vi "create buffer exchange.vi"(6 "FIFO modes (polling)":T2, 8 "error in":errorcluster, 10 "buffer count":u16, 11 "initial data table":T3) -> (0 "error out":errorcluster, 2 "consumer":T1, 3 "producer":T1)   [LabVIEW 2013, in "tag bus buffer exchange.lvlib"]
uses:
  tag bus buffer exchange.lvlib
  table/data table.ctl
  buffer exchange.ctl
  buffer reference.ctl
  table/data table.lvlib
  tag bus.lvlib
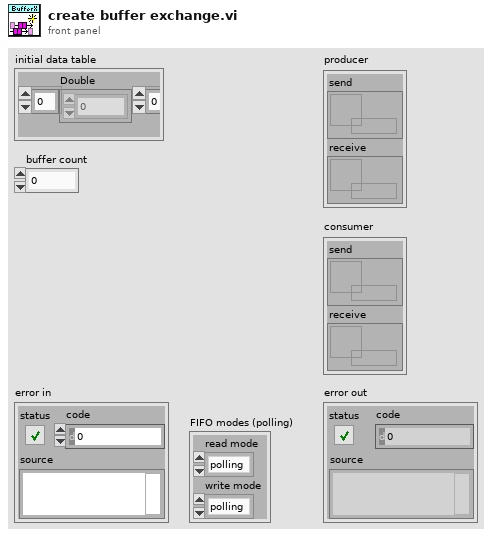
[diagram p1: front panel]
types:
  T1 = typedef "tag bus buffer exchange.lvlib/buffer exchange.ctl" = cluster{"send":refnum<k33>, "receive":refnum<k33>}
  T2 = cluster{"read mode":enum16{"polling", "blocking"}, "write mode":enum16{"polling", "blocking"}}
  T3 = typedef "tag bus.lvlib/data table.lvlib/data table.ctl" = cluster{"Double":dbl[], "Single":sgl[], "I64":i64[], "I32":i32[], "I16":i16[], "I8":i8[], "U64":u64[], "U32":u32[], "U16":u16[], "U8":u8[], "Boolean":bool[], "String":string[], "Array of Double":cluster{"DBL Array":dbl[]}[], "Array of Single":cluster{"SGL Array":sgl[]}[], "Array of I64":cluster{"I64 Array":i64[]}[], "Array of I32":cluster{"I32 Array":i32[]}[], "Array of I16":cluster{"I16 Array":i16[]}[], "Array of I8":cluster{"I8 Array":i8[]}[], "Array of U64":cluster{"U64 Array":u64[]}[], "Array of U32":cluster{"U32 Array":u32[]}[], "Array of U16":cluster{"U16 Array":u16[]}[], "Array of U8":cluster{"U8 Array":u8[]}[], "Array of Boolean":cluster{"Boolean Array":bool[]}[], "Array of String":cluster{"String Array":string[]}[]}
  T4 = typedef "tag bus buffer exchange.lvlib/buffer reference.ctl" = refnum<data-value>
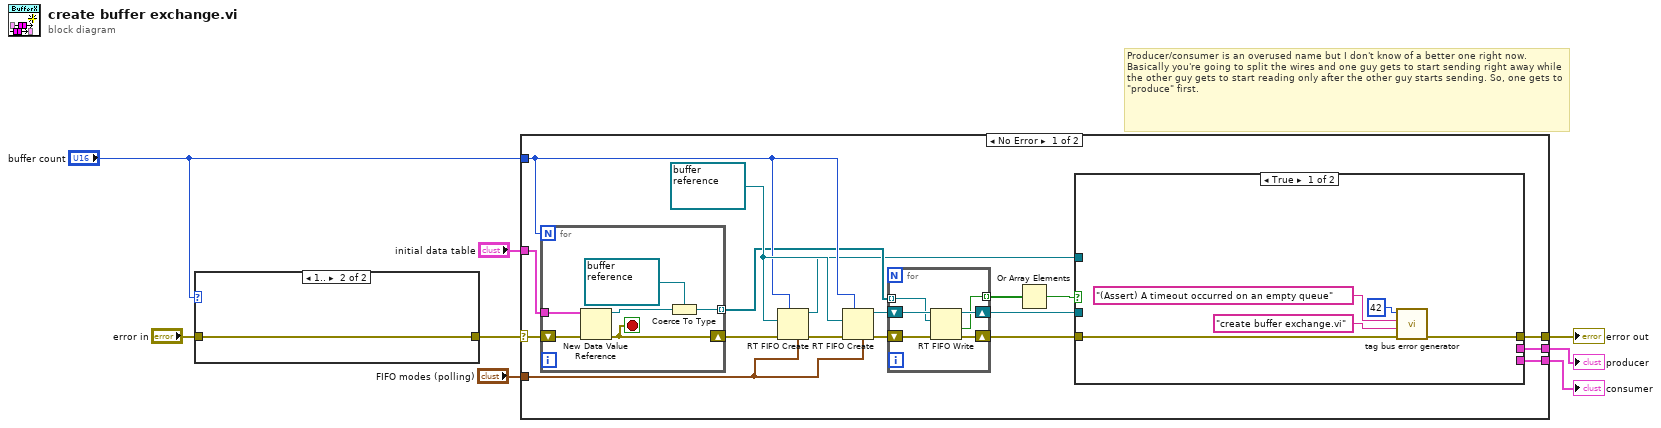
[diagram p0: block diagram]
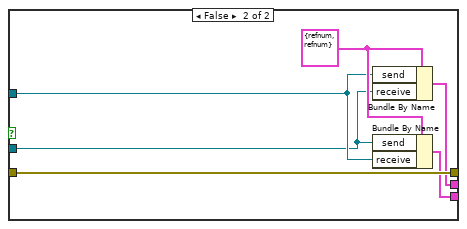
[diagram p2: hidden frame]
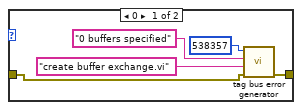
[diagram p4: hidden frame]
diagram:
  # "Producer/consumer is an overused name but I don't know of a better one right now. Basically you're going to split the wires and one guy gets to start sending right away while the other guy gets to start reading only after the other guy starts sending. So, one gets to \"produce\" first."
  n1 = case shown="1.." "buffer count" {
    tunnel: [w9 w14] -> w7
    tunnel: "error in" -> [w12 w14]
    frame 0 {
      n2 = call "tag bus error generator.vi"("error in"=w12, "source"="create buffer exchange.vi", "append error message"="0 buffers specified", "error code (0)"=538357) -> ("error out"=w9:errorcluster)  [unwired: 5 in]
    }
    frame 1.. {
    }
  }
  n3 = case shown="No Error" w7 {
    selector: w7 -> [w32 w56]
    tunnel: [w19 w56] -> w6
    tunnel: [w18 _] -> w5
    tunnel: "buffer count" -> [w25 _]
    tunnel: "initial data table" -> [w31 _]
    tunnel: "FIFO modes (polling)" -> [w27 _]
    tunnel: [w17 _] -> w1
    frame No Error {
      w28 = T4 refnum ("buffer")
      n4 = for {
        N: w25 -> [_]
        shift-right: [w54] -> w30
        shift-left: w32 -> [w55]
        tunnel: w31 -> [w53]
        tunnel: [w51] -> w23 mode=indexing
        stop <- w54 stop-if-true
        n5 = New Data Value Reference(data value=w53, error in=w55) -> (data value reference=w52:refnum<data-value>, error out=w54:errorcluster)
        n6 = Coerce To Type(0:w52, 1:T4 refnum ("buffer")) -> (2:w51:T4)
      }
      n7 = RT FIFO Create(1:w28, 3:w30, 4:w25, 7:w27) -> (8:w15:refnum<k33>, 11:w29:errorcluster)  [unwired: 4 in, 1 out]
      n8 = RT FIFO Create(1:w28, 3:w29, 4:w25, 7:w27) -> (8:w24:refnum<k33>, 11:w26:errorcluster)  [unwired: 4 in, 1 out]
      n9 = for {
        shift-right: [w47] -> w16
        shift-left: w24 -> [w49]
        shift-right: [w46] -> w20
        shift-left: w26 -> [w48]
        tunnel: w23 -> [w45] mode=indexing
        tunnel: [w44] -> w22 mode=indexing
        n10 = RT FIFO Write(0:w49, 1:w45, 3:w48) -> (8:w47:refnum<k33>, 10:w44:bool, 11:w46:errorcluster)  [unwired: 2 in, 1 out]
      }
      n11 = Or Array Elements(Boolean array=w22) -> (logical OR=w21:bool)
      n12 = case shown="True" w21 {
        tunnel: [w33 w43] -> w19
        tunnel: w20 -> [w36 w43]
        tunnel: [_ w41] -> w18
        tunnel: [_ w40] -> w17
        tunnel: w16 -> [_ w38]
        tunnel: w15 -> [_ w39]
        frame True {
          n13 = call "tag bus error generator.vi"("error in"=w36, "source"="create buffer exchange.vi", "append error message"="(Assert) A timeout occurred on an empty queue", "error code (0)"=42) -> ("error out"=w33:errorcluster)  [unwired: 5 in]
        }
        frame False {
          w42 = T1 {"send"=refnum, "receive"=refnum} ("buffer exchange")
          n14 = Bundle By Name(cluster=w42, "send"=w39, "receive"=w38) -> (w41:T1)
          n15 = Bundle By Name(cluster=w42, "send"=w38, "receive"=w39) -> (w40:T1)
        }
      }
    }
    frame Error {
    }
  }
  "error out" <- w6
  "producer" <- w5
  "consumer" <- w1
